vi "VI-Find Terminals.vi"(0 "VI in":refnum<vi>, 2 "Traverse Target":T1=enum."BD", 5 "Class Name":string="ControlTerminal", 7 "Names":string[](array[string]), 11 "error in (no error)":errorcluster) -> (4 "VI out":refnum<vi>, 8 "Array":refnum<vi>[](array[refnum]), 15 "error out":errorcluster)   [LabVIEW 2015]
uses:
  <vilib>/Utility/traverseref.llb/TRef TravTarget.ctl
  <vilib>/Utility/traverseref.llb/VI Scripting - Traverse.lvlib
panel:
  out "Array 2":string[](array[string])
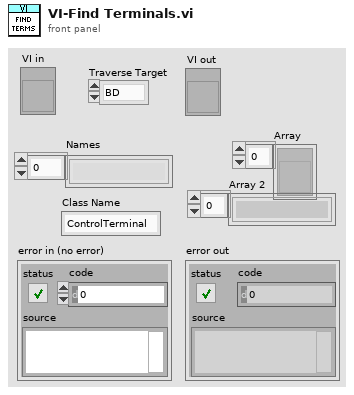
[diagram p1: front panel]
types:
  T1 = typedef "TRef TravTarget.ctl" = enum16{"FP", "BD", "Other"}
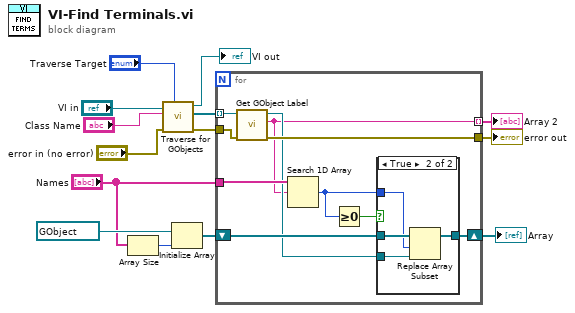
[diagram p0: block diagram]
diagram:
  n1 = Array Size(array="Names") -> (size(s)=w6:i32)
  n2 = call <vilib>:"Traverse for GObjects.vi"("Traverse Target"="Traverse Target", "error in (no error)"="error in (no error)", "Class Name"="Class Name", "VI Refnum"="VI in") -> ("error out"=w9:errorcluster, "References"=w13:refnum<vi>[], "dup VI Refnum"=→"VI out":refnum<vi>)  [unwired: 4 in, 1 out]
  n3 = Initialize Array(refnum<vi> refnum ("dup GObject"), w6) -> (w4:refnum<vi>[])
  n4 = for {
    tunnel: w13 -> [w15] mode=indexing
    tunnel: w9 -> [w24]
    tunnel: "Names" -> [w23]
    tunnel: [w22] -> w8
    shift-right: [w18] -> w3
    shift-left: w4 -> [w21]
    tunnel: [w16] -> w1 mode=indexing
    n5 = call <vilib>:"Get GObject Label.vi"("error in (no error)"=w24, "GObject"=w15) -> ("error out"=w22:errorcluster, "Object Label"=w16:string, "dup GObject"=w17:refnum<vi>)  [unwired: 5 in, 2 out]
    n6 = Search 1D Array(1D array=w23, element=w16) -> (index of element=w19:i32)  [unwired: 1 in]
    n7 = Greater Or Equal To 0?(x=w19) -> (x >= 0?=w20:bool)
    n8 = case shown="True" w20 {
      tunnel: w21 -> [w25 w29]
      tunnel: w19 -> [_ w28]
      tunnel: [w25 w27] -> w18
      tunnel: w17 -> [_ w26]
      frame False {
      }
      frame True {
        n9 = Replace Array Subset(array=w29, new element=w26, index=w28) -> (w27:refnum<vi>[])
      }
    }
  }
  "error out" <- w8
  "Array" <- w3
  "Array 2" <- w1
